vi "Add Rx Monitor Section and Status Channels.vi"(8 "error in":errorcluster, 11 "port ref in":T1 format="%.0x") -> (0 "error out":errorcluster, 1 "Rx monitor channel refs":T1[](array[typedef]) format="%.0x", 2 "Rx monitor ref out":T1 format="%.0x", 3 "port ref out":T1 format="%.0x")   [LabVIEW 2020, in "AIM ARINC 664 Scripting.lvlib"]
uses:
  AIM ARINC 664 Scripting.lvlib
  <vilib>/NI VeriStand/Custom Device API/Custom Device Item Ref.ctl
  <vilib>/NI VeriStand/Custom Device API/Custom Device Channel.ctl
  <vilib>/NI VeriStand/Custom Device API/Custom Device Channel Type.ctl
  Constants.vi
  <vilib>/NI VeriStand/Custom Device API/Custom Device API.lvlib
  <vilib>/Utility/Data Type/NI_Data Type.lvlib
  <vilib>/NI/NI VeriStand Advanced SysDef API/SysDef API/Advanced System Definition.lvlib
  Shared/RxStatus Enum.ctl
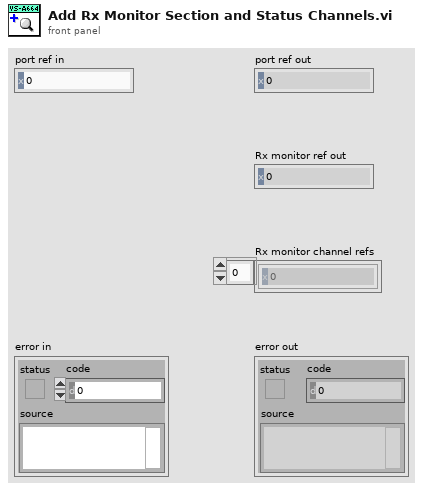
[diagram p1: front panel]
types:
  T1 = typedef "Custom Device API.lvlib/Custom Device Item Ref.ctl" = u64
  T2 = enum16{"FDX_MON_STAT_EMPTY", "FDX_MON_STAT_FILLED", "FDX_MON_STAT_FULL", "FDX_MON_STAT_OVERFLOW", "FDX_MON_STAT_ERROR"}
  T3 = typedef "RxStatus Enum.ctl" = enum16{"FDX_STAT_STOP", "FDX_STAT_RUN", "FDX_STAT_ERROR"}
  T4 = typedef "Custom Device API.lvlib/Custom Device Channel.ctl" = cluster{"Type":T5, "Units":string, "Default Value":dbl, "Faultable":bool, "Scalable":bool}
  T5 = typedef "Custom Device API.lvlib/Custom Device Channel Type.ctl" = enum16{"Input", "Output"}
  T6 = enum16{"FDX_STAT_STOP", "FDX_STAT_RUN", "FDX_STAT_ERROR"}
  T7 = cluster{"Monitor Reset Mode":string, "enum names":string[], "Values":dbl[]}
  T8 = cluster{"Monitor QueueStatus Channel":string, "enum names":string[], "Values":dbl[]}
  T9 = cluster{"Monitor RxStatus Channel":string, "enum names":string[], "Values":dbl[]}
  T10 = cluster{"Monitor Reset Mode":string, "enum names":string[], "Values":dbl[]}[]
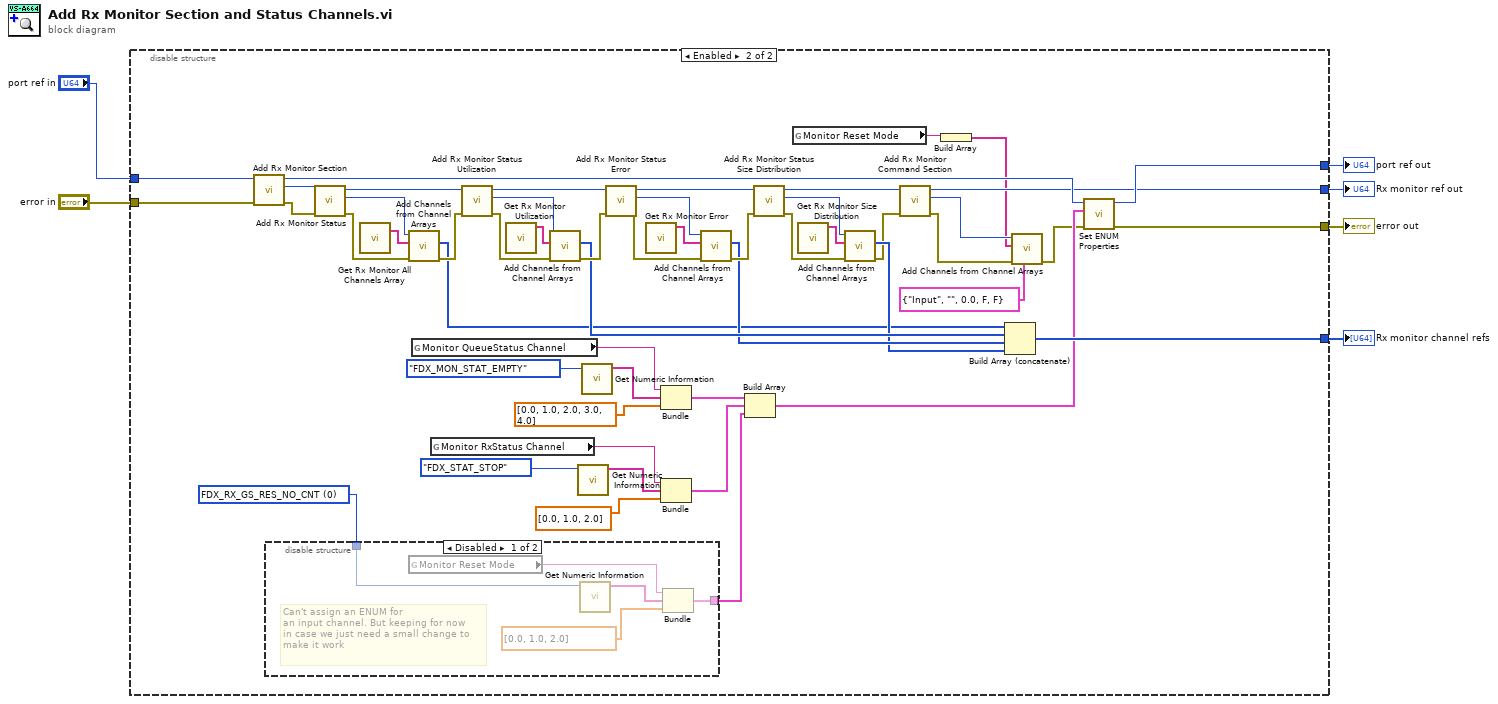
[diagram p0: block diagram]
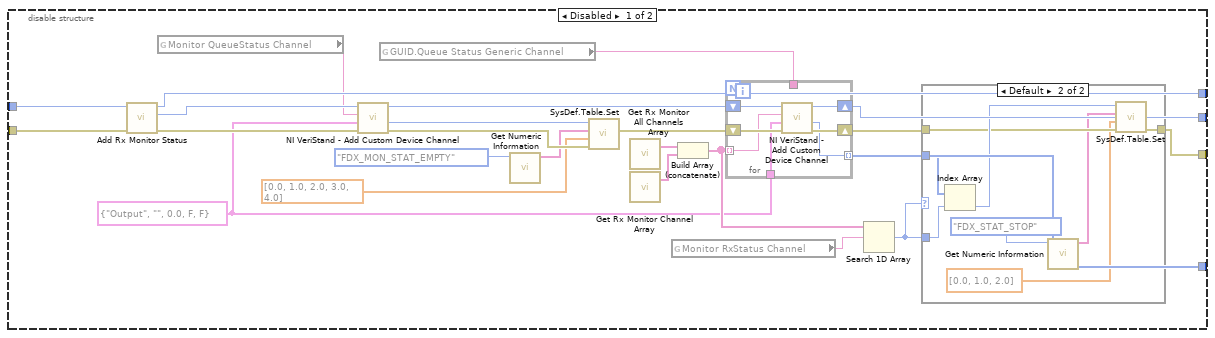
[diagram p2: hidden frame]
diagram:
  n1 = disable-structure shown="Enabled" {
    disable-tunnel: "port ref in" -> [w30 w98]
    disable-tunnel: "error in" -> [w29 w97]
    disable-tunnel: [w27 w54] -> w4
    disable-tunnel: [w26 w66] -> w3
    disable-tunnel: [w11 w80] -> w2
    disable-tunnel: [w8 w75] -> w1
    frame Disabled {
      w7 = T4 {"Type"=enum."Output", "Units"="", "Default Value"=0.0, "Faultable"=FALSE, "Scalable"=FALSE} ("Channel")
      n2 = call "Add Rx Monitor Status.vi"("error in (no error)"=w29, "Rx monitor ref in"=w30) -> ("error out"=w28:errorcluster, "Rx monitor status ref out"=w25:T1, "Rx monitor ref out"=w26:T1)  [unwired: 7 in]
      n3 = global read "Constants.vi" "Monitor QueueStatus Channel"() -> (w24:string)
      n4 = call <vilib>:"NI VeriStand - Add Custom Device Channel.vi"("error in (no error)"=w28, "Channel"=w7, "Channel Name"=w24, "Parent Ref in"=w25) -> ("error out"=w21:errorcluster, "Channel Ref"=w19:T1, "Parent Ref out"=w22:T1)  [unwired: 4 in, 1 out]
      n5 = global read "Constants.vi" "GUID.Queue Status Generic Channel"() -> (w23:string)
      n6 = call <vilib>:"Get Numeric Information.vi"("variant"=T2."FDX_MON_STAT_EMPTY" ("Enum")) -> ("enum names"=w18:string[])  [unwired: 7 in, 3 out]
      n7 = call <vilib>:"SysDef.Table.Set.vi"("error in (no error)"=w21, "Values"=dbl[] [0.0, 1.0, 2.0, 3.0, 4.0], "Names"=w18, "nodeID"=w19) -> ("error out"=w20:errorcluster)  [unwired: 6 in, 1 out]
      n8 = call "Get Rx Monitor All Channels Array.vi"() -> ("channel array"=w15:string[])  [unwired: 3 in]
      n9 = call "Get Rx Monitor Channel Array.vi"() -> ("channel array"=w14:string[])  [unwired: 3 in]
      n10 = global read "Constants.vi" "Monitor RxStatus Channel"() -> (w13:string)
      n11 = Build Array (concatenate)(w15, w14) -> (w12:string[])
      n12 = for {
        tunnel: [w42] -> w11 mode=indexing
        shift-right: [w43] -> w9
        shift-left: w20 -> [w46]
        tunnel: w12 -> [w40] mode=indexing
        tunnel: w7 -> [w41]
        tunnel: w23 -> [_]
        shift-right: [w45] -> w27
        shift-left: w22 -> [w44]
        n13 = call <vilib>:"NI VeriStand - Add Custom Device Channel.vi"("error in (no error)"=w46, "Channel"=w41, "Channel Name"=w40, "Parent Ref in"=w44) -> ("error out"=w43:errorcluster, "Channel Ref"=w42:T1, "Parent Ref out"=w45:T1)  [unwired: 4 in, 1 out]
      }
      n14 = Search 1D Array(1D array=w12, element=w13) -> (index of element=w10:i32)  [unwired: 1 in]
      n15 = case shown="Default" w10 {
        tunnel: w11 -> [_ w39]
        tunnel: w10 -> [_ w38]
        tunnel: w9 -> [w31 w36]
        tunnel: [w31 w35] -> w8
        frame -1 {
        }
        frame Default {
          n16 = Index Array(array=w39, index=w38) -> (element=w37:T1)
          n17 = call <vilib>:"Get Numeric Information.vi"("variant"=RxStatus_Enum."FDX_STAT_STOP" ("Enum")) -> ("enum names"=w33:string[])  [unwired: 7 in, 3 out]
          n18 = call <vilib>:"SysDef.Table.Set.vi"("error in (no error)"=w36, "Values"=dbl[] [0.0, 1.0, 2.0], "Names"=w33, "nodeID"=w37) -> ("error out"=w35:errorcluster)  [unwired: 6 in, 1 out]
        }
      }
    }
    frame Enabled {
      w47 = u32 0 items=["FDX_RX_GS_RES_NO_CNT", "FDX_RX_GS_RES_ALL_CNT", "FDX_RX_GS_RES_ERR_CNT"] ("Control")
      n19 = call "Add Rx Monitor Section.vi"("error in"=w97, "port ref in"=w98) -> ("error out"=w62:errorcluster, "Rx monitor ref out"=w65:T1, "port ref out"=w67:T1)  [unwired: 7 in]
      n20 = disable-structure shown="Disabled" {
        disable-tunnel: [w101 _] -> w57
        disable-tunnel: w47 -> [w99 _]
        frame Disabled {
          # "Can't assign an ENUM for \nan input channel. But keeping for now\nin case we just need a small change to\nmake it work"
          n21 = global read "Constants.vi" "Monitor Reset Mode"() -> (w100:string)
          n22 = call <vilib>:"Get Numeric Information.vi"("variant"=w99) -> ("enum names"=w103:string[])  [unwired: 7 in, 3 out]
          n23 = Bundle("Monitor Reset Mode"=w100, "enum names"=w103, "Values"=dbl[] [0.0, 1.0, 2.0]) -> (w101:T7)  [unwired: 1 in]
        }
        frame Enabled {
        }
      }
      n24 = call "Add Rx Monitor Status.vi"("error in (no error)"=w62, "Rx monitor ref in"=w65) -> ("error out"=w61:errorcluster, "Rx monitor status ref out"=w64:T1, "Rx monitor ref out"=w63:T1)  [unwired: 7 in]
      n25 = call "Get Rx Monitor All Channels Array.vi"() -> ("channel array"=w78:string[])  [unwired: 3 in]
      n26 = call "Add Channels from Channel Arrays.vi"("error in"=w61, "channel array"=w78, "section ref in"=w64) -> ("error out"=w79:errorcluster, "channel refs"=w60:T1[])  [unwired: 6 in, 1 out]
      n27 = global read "Constants.vi" "Monitor QueueStatus Channel"() -> (w58:string)
      n28 = global read "Constants.vi" "Monitor RxStatus Channel"() -> (w59:string)
      n29 = call "Add Rx Monitor Status Utilization.vi"("error in (no error)"=w79, "Rx monitor ref in"=w63) -> ("error out"=w85:errorcluster, "Rx monitor status utilitzation ref out"=w84:T1, "Rx monitor ref out"=w87:T1)  [unwired: 7 in]
      n30 = call "Get Rx Monitor Utilization.vi"() -> ("channel array"=w86:string[])  [unwired: 11 in]
      n31 = call "Add Channels from Channel Arrays.vi"("error in"=w85, "channel array"=w86, "section ref in"=w84) -> ("error out"=w88:errorcluster, "channel refs"=w83:T1[])  [unwired: 6 in, 1 out]
      n32 = call <vilib>:"Get Numeric Information.vi"("variant"=T6."FDX_STAT_STOP" ("Enum")) -> ("enum names"=w71:string[])  [unwired: 7 in, 3 out]
      n33 = call <vilib>:"Get Numeric Information.vi"("variant"=T2."FDX_MON_STAT_EMPTY" ("Enum")) -> ("enum names"=w74:string[])  [unwired: 7 in, 3 out]
      n34 = call "Add Rx Monitor Status Error.vi"("error in (no error)"=w88, "Rx monitor ref in"=w87) -> ("error out"=w92:errorcluster, "Rx monitor status error ref out"=w89:T1, "Rx monitor ref out"=w94:T1)  [unwired: 7 in]
      n35 = call "Get Rx Monitor Error.vi"() -> ("channel array"=w96:string[])  [unwired: 11 in]
      n36 = Bundle("Monitor QueueStatus Channel"=w58, "enum names"=w74, "Values"=dbl[] [0.0, 1.0, 2.0, 3.0, 4.0]) -> (w69:T8)  [unwired: 1 in]
      n37 = Bundle("Monitor RxStatus Channel"=w59, "enum names"=w71, "Values"=dbl[] [0.0, 1.0, 2.0]) -> (w70:T9)  [unwired: 1 in]
      n38 = call "Add Channels from Channel Arrays.vi"("error in"=w92, "channel array"=w96, "section ref in"=w89) -> ("error out"=w93:errorcluster, "channel refs"=w82:T1[])  [unwired: 6 in, 1 out]
      n39 = Build Array(w69, w70, w57) -> (w68:T10)
      n40 = call "Add Rx Monitor Status Size Distribution.vi"("error in (no error)"=w93, "Rx monitor ref in"=w94) -> ("error out"=w90:errorcluster, "Rx monitor size distribution ref out"=w91:T1, "Rx monitor ref out"=w56:T1)  [unwired: 7 in]
      n41 = global read "Constants.vi" "Monitor Reset Mode"() -> (w50:string)
      n42 = call "Get Rx Monitor Size Distribution.vi"() -> ("channel array"=w95:string[])  [unwired: 11 in]
      n43 = call "Add Channels from Channel Arrays.vi"("error in"=w90, "channel array"=w95, "section ref in"=w91) -> ("error out"=w55:errorcluster, "channel refs"=w81:T1[])  [unwired: 6 in, 1 out]
      n44 = call "Add Rx Monitor Command Section.vi"("error in"=w55, "Tx generic ref in"=w56) -> ("error out"=w52:errorcluster, "Tx generic command section ref out"=w53:T1, "Tx generic ref out"=w54:T1)  [unwired: 7 in]
      n45 = Build Array(w50) -> (w49:string[])
      n46 = Build Array (concatenate)(w60, w83, w82, w81) -> (w80:T1[])
      n47 = call "Add Channels from Channel Arrays.vi"("Channel"=T4 {"Type"=enum."Input", "Units"="", "Default Value"=0.0, "Faultable"=FALSE, "Scalable"=FALSE}, "error in"=w52, "channel array"=w49, "section ref in"=w53) -> ("error out"=w51:errorcluster)  [unwired: 5 in, 2 out]
      n48 = call "Set ENUM Properties.vi"("error in"=w51, "enum to be changes"=w68, "parent ref in"=w67) -> ("error out"=w75:errorcluster, "parent ref out"=w66:T1)  [unwired: 7 in]
    }
  }
  "Rx monitor ref out" <- w4
  "port ref out" <- w3
  "error out" <- w1
  "Rx monitor channel refs" <- w2
